vi "SaveComicCache.vi"(8 "error in (no error)":errorcluster, 11 "Comics in":refnum<class "Comics.lvclass">) -> (0 "error out":errorcluster, 3 "Comics out":refnum<class "Comics.lvclass">)   [LabVIEW 2022 SP3, in "Comics.lvclass"]
uses:
  Comics.lvclass
  Comics.lvclass/Comics.ctl
  <vilib>/Utility/cursorutil.llb/Set Cursor (Icon Pict).vi
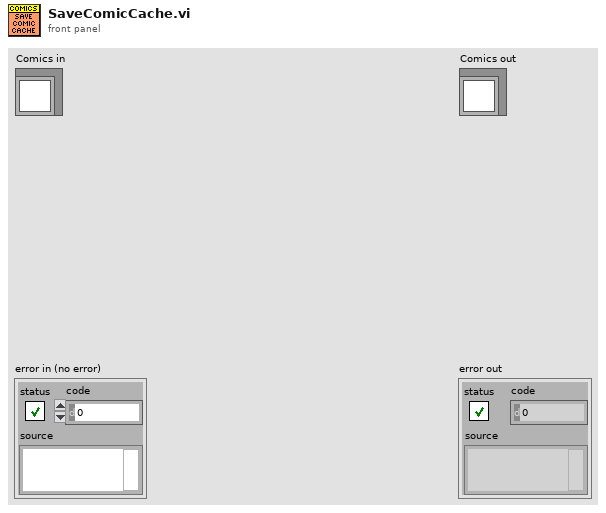
[diagram p1: front panel]
types:
  T1 = typedef "Comic.ctl" = cluster{"URL":string, "Series URL":string, "Series":string, "Volume":i32, "Issue":string, "Title":string, "Description":string, "Page Count":i32, "Cover Price":dbl, "UPC":string, "Characters":T2[], "Creators":T3[], "Main Cover URL":string, "Variant Covers":T4[], "DatePublished":timestamp}
  T2 = typedef "Character.ctl" = cluster{"Name":string, "Real-Name":string, "Universe":string, "URL":string}
  T3 = typedef "Creator.ctl" = cluster{"Name":string, "URL":string, "Creator Types":string[]}
  T4 = typedef "Variant.ctl" = cluster{"URL":string, "Description":string, "Cover URL":string}
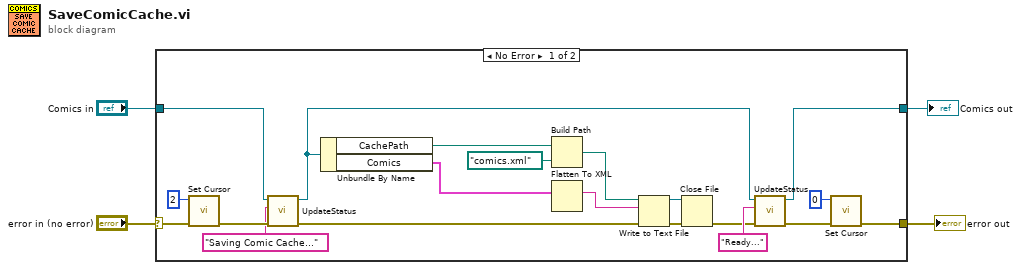
[diagram p0: block diagram]
diagram:
  n1 = case shown="No Error" "error in (no error)" {
    selector: "error in (no error)" -> [w17 w26]
    tunnel: [w16 w26] -> w3
    tunnel: [w8 w25] -> w1
    tunnel: "Comics in" -> [w15 w25]
    frame No Error {
      n2 = call-poly <vilib>:"Set Cursor.vi"("error in (no error)"=w17, "icon"=u16 2) -> ("error out"=w14:errorcluster)  [unwired: 8 in, 1 out]
      n3 = call "UpdateStatus.vi"("error in (no error)"=w14, "Status"="Saving Comic Cache...", "Comics in"=w15) -> ("error out"=w13:errorcluster, "Comics out"=w9:refnum<class "Comics.lvclass">)  [unwired: 7 in]
      n4 = Unbundle By Name(w9) -> ("CachePath"=w24:path, "Comics"=w22:T1[])
      n5 = Build Path(base path=w24, name or relative path=path "comics.xml") -> (appended path=w20:path)
      n6 = Flatten To XML(6:w22) -> (2:w21:string)
      n7 = Write to Text File(file (use dialog)=w20, text=w21, error in=w13) -> (refnum out=w18:refnum<file>, error out=w19:errorcluster)  [unwired: 1 in, 1 out]
      n8 = Close File(refnum=w18, error in=w19) -> (error out=w10:errorcluster)  [unwired: 1 out]
      n9 = call "UpdateStatus.vi"("error in (no error)"=w10, "Status"="Ready...", "Comics in"=w9) -> ("error out"=w7:errorcluster, "Comics out"=w8:refnum<class "Comics.lvclass">)  [unwired: 7 in]
      n10 = call-poly <vilib>:"Set Cursor.vi"("error in (no error)"=w7, "icon"=u16 0) -> ("error out"=w16:errorcluster)  [unwired: 8 in, 1 out]
    }
    frame Error {
    }
  }
  "error out" <- w3
  "Comics out" <- w1
